vi "Check If Folder Exists.vi"(11 "Folder Path":path) -> (3 "Valid Folder?":bool)   [LabVIEW 2026, in "NIVS_CDEW_MetaDataObj.lvclass"]
uses:
  NIVS_CDEW_MetaDataObj.lvclass
  NIVS_CDEW_MetaDataObj.lvclass/NIVS_CDEW_MetaDataObj.ctl
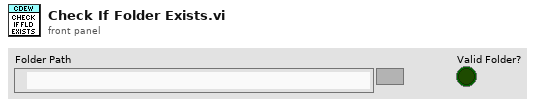
[diagram p1: front panel]
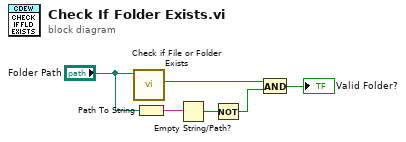
[diagram p0: block diagram]
diagram:
  n1 = call <vilib>:"Check if File or Folder Exists.vi"("path"="Folder Path") -> ("file or folder exists?"=w3:bool)  [unwired: 8 in, 2 out]
  n2 = Path To String(path="Folder Path") -> (string=w6:string)
  n3 = Empty String/Path?(string/path=w6) -> (empty?=w5:bool)
  n4 = Not(x=w5) -> (.not. x?=w4:bool)
  n5 = And(x=w3, y=w4) -> (x .and. y?=→"Valid Folder?":bool)
